vi "Run-Time Menu - Remove Module Entry--helper.vi"(7 "Menu in":refnum<k9>, 8 "error in":errorcluster, 11 "Module DQMH Path":path) -> (0 "error out":errorcluster)   [LabVIEW 2022 SP3, in "UI Manager.lvlib"]
doc: "____\nHAMPEL SOFTWARE ENGINEERING v2.6.0 (2023-12-19 10:54)"
uses:
  UI Manager.lvlib
  <vilib>/Hampel Software Engineering/HSE Logger/hse-logger.lvlib
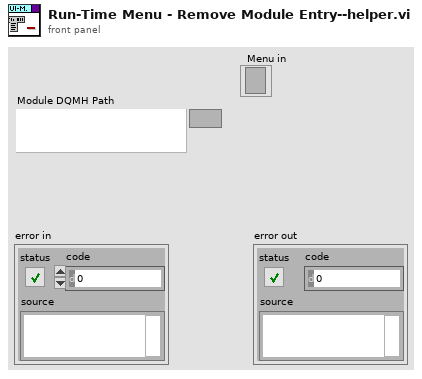
[diagram p1: front panel]
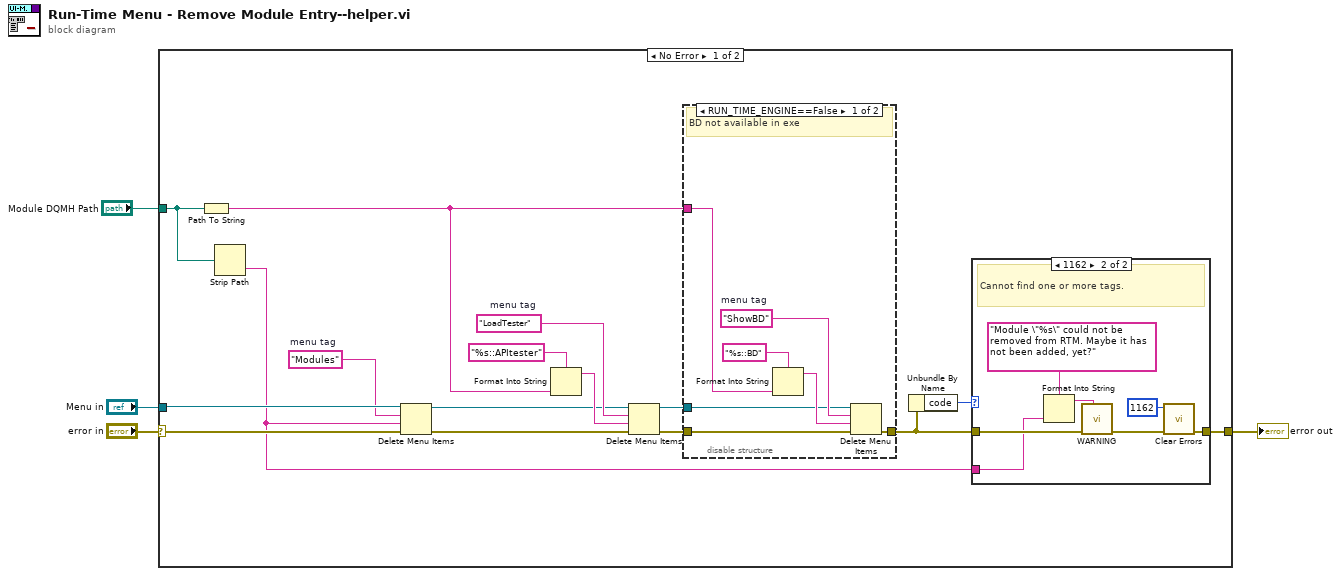
[diagram p0: block diagram]
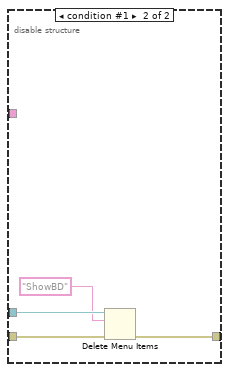
[diagram p3: hidden frame]
diagram:
  n1 = case shown="No Error" "error in" {
    selector: "error in" -> [w20 w40]
    tunnel: [w8 w40] -> w4
    tunnel: "Module DQMH Path" -> [w11 _]
    tunnel: "Menu in" -> [w19 _]
    frame No Error {
      w13 = "Modules"  # menu tag
      w16 = "LoadTester"  # menu tag
      n2 = Path To String(path=w11) -> (string=w10:string)
      n3 = Strip Path(path=w11) -> (name=w5:string)  [unwired: 1 out]
      n4 = Delete Menu Items(6:w20, 7:w5, 8:w13, 9:w19) -> (0:w9:errorcluster, 3:w12:refnum<k9>)
      n5 = Format Into String(format string="%s::APItester", w10) -> (resulting string=w18:string)  [unwired: 2 in, 1 out]
      n6 = Delete Menu Items(6:w9, 7:w18, 8:w16, 9:w12) -> (0:w14:errorcluster, 3:w15:refnum<k9>)
      n7 = disable-structure shown="RUN_TIME_ENGINE==False" {
        disable-tunnel: w15 -> [w29 w39]
        disable-tunnel: w14 -> [w34 w38]
        disable-tunnel: [w35 w37] -> w7
        disable-tunnel: w10 -> [w30 _]
        frame condition #0 (active) {
          w33 = "ShowBD"  # menu tag
          # "BD not available in exe"
          n8 = Format Into String(format string="%s::BD", w30) -> (resulting string=w31:string)  [unwired: 2 in, 1 out]
          n9 = Delete Menu Items(6:w34, 7:w31, 8:w33, 9:w29) -> (0:w35:errorcluster)  [unwired: 1 out]
        }
        frame condition #1 {
          n10 = Delete Menu Items(6:w38, 8:"ShowBD" ("menu tag"), 9:w39) -> (0:w37:errorcluster)  [unwired: 1 in, 1 out]
        }
      }
      n11 = Unbundle By Name(w7) -> ("code"=w6:i32)
      n12 = case shown="1162" w6 {
        tunnel: [w21 w27] -> w8
        tunnel: w7 -> [w21 w26]
        tunnel: w5 -> [_ w22]
        frame 0, Default {
        }
        frame 1162 {
          # "Cannot find one or more tags."
          n13 = Format Into String(format string="Module \"%s\" could not be removed from RTM. Maybe it has not been added, yet?", w22) -> (resulting string=w24:string)  [unwired: 2 in, 1 out]
          n14 = call <vilib>:"WARNING.vi"("Message"=w24, "error in"=w26) -> ("error out"=w25:errorcluster)  [unwired: 9 in]
          n15 = call <vilib>:"Clear Errors.vi"("error in (no error)"=w25, "specific error code to clear (0: all)"=1162) -> ("error out"=w27:errorcluster)  [unwired: 4 in, 1 out]
        }
      }
    }
    frame Error {
    }
  }
  "error out" <- w4
